vi "LVRT Serial Init.vi"(6 "stop bits (10: 1 bit)":u16(ring)=10 items=["1 bit"=10, "1.5 bits"=15, "2 bits"=20], 7 "Invert Polarity?":bool, 8 "error in (no error)":errorcluster, 9 "parity (0:none)":u16(ring) items=["None", "Odd", "Even", "Mark", "Space"], 10 "data bits (8)":u16=8 min=5 max=8 step=1, 11 "baud rate (9600)":u32=543478) -> (0 "error out":errorcluster, 3 "FPGA VI Reference Out":T1)   [LabVIEW 2009]
uses:
  serial FPGA main reference type def.ctl
  <vilib>/rvi/interface/nirviOpenFPGA/nirviOpenFPGA.xnode
  FPGA Bitfiles/Athena Brain.lvproj_FPGA Target 2_serial FPGA Main.vi.lvbitx
  serial FPGA Main.vi
  <vilib>/FPGAPlugInAG/sbRIO-9642/nirviIntfOpen_sbRIO-9642.vi
  <vilib>/rvi/interface/nirviReadWriteControl/nirviReadWriteControl.xnode
  <vilib>/Utility/error.llb/Error Cluster From Error Code.vi
  <vilib>/rvi/errors/niLvFpgaAdjustHostInterfaceError.vi
  <vilib>/rvi/interface/common/niFpgaNodeNameForErrorReporting.ctl
  <vilib>/rvi/errors/niLvFpgaWhatHappensToTopLevelVI.ctl
  <vilib>/rvi/interface/nirviMethod/nirviMethod.xnode
  <vilib>/RVI Host/nirviSupport.llb/nirviErrorClusterFromErrorCode.vi
  <vilib>/LabVIEW Targets/FPGA/RIO/nirio_HostInterface/nirio_EnableInterrupts.vi
  <vilib>/rvi/errors/niLvFpgaReportInternalErrorWithAdditionalInfo.vi
  <vilib>/userDefined/High Color/nirio_resource_hc.ctl
  NiRioSrv.dll
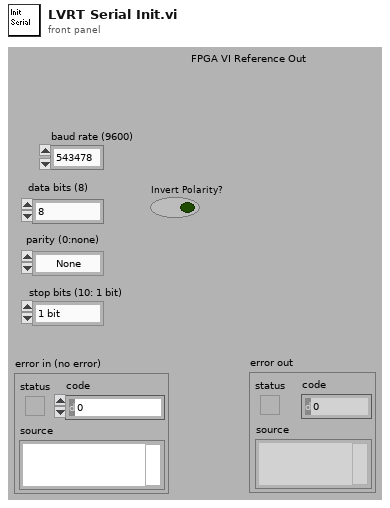
[diagram p1: front panel]
types:
  T1 = typedef "serial FPGA main reference type def.ctl" = refnum<k20>
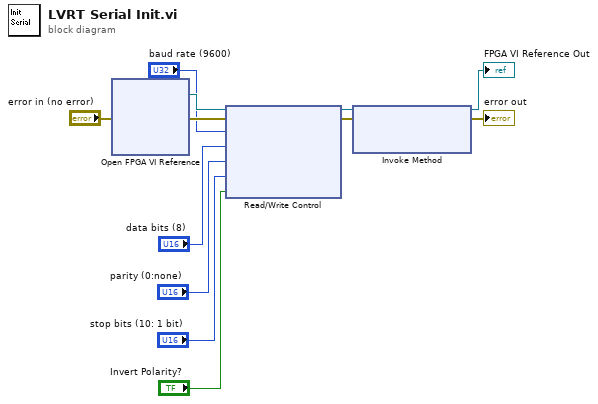
[diagram p0: block diagram]
diagram:
  n1 = xnode "Open FPGA VI Reference"("error in"="error in (no error)") -> ("FPGA VI Reference Out"=w12:refnum<k20>, "error out"=w11:errorcluster)  [unwired: 1 in]
  n2 = xnode "Read/Write Control"("FPGA VI Reference In"=w12, "error in"=w11, "baud rate (9600)"="baud rate (9600)", "data bits (8)"="data bits (8)", "parity (0:none)"="parity (0:none)", "stop bits (10: 1 bit)"="stop bits (10: 1 bit)", "Invert Polarity?"="Invert Polarity?") -> ("FPGA VI Reference Out"=w6:refnum<k20>, "error out"=w5:errorcluster)
  n3 = xnode "Invoke Method"("FPGA VI Reference In"=w6, "error in"=w5) -> ("FPGA VI Reference Out"=→"FPGA VI Reference Out":refnum<k20>, "error out"=→"error out":errorcluster)  [unwired: 1 out]
